vi "(Depricated) Nitrogen Feed Core.vi"() -> ()   [LabVIEW 2015]
doc: "Reads Storage Line State variable. Opens a single line."
panel:
  in  "error in (no error)":errorcluster
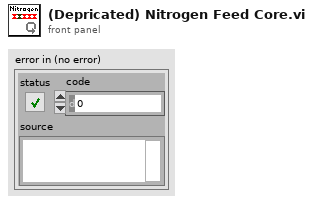
[diagram p1: front panel]
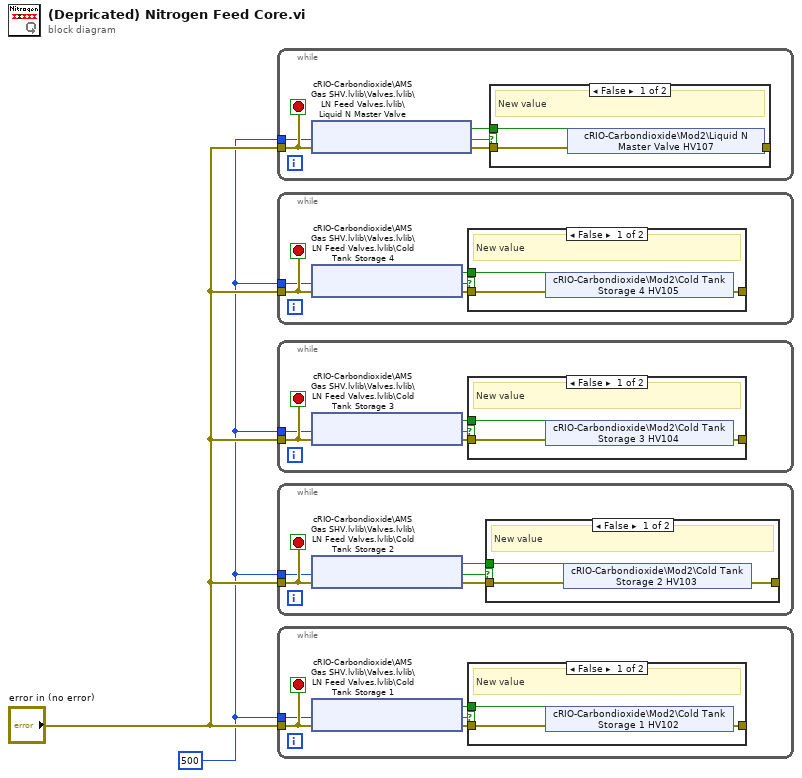
[diagram p0: block diagram]
diagram:
  w1 = 500 ("ms timeout (0)")
  n1 = while {
    tunnel: "error in (no error)" -> [w4]
    tunnel: w1 -> [w3]
    stop <- w4 stop-if-true
    n2 = shared-variable "cRIO-Carbondioxide\\AMS Gas SHV.lvlib\\Valves.lvlib\\LN Feed Valves.lvlib\\Liquid N Master Valve"(error in=w4, w3) -> (w5:bool, error out=w7:errorcluster, w6:bool)
    n3 = case shown="False" w6 {
      tunnel: w7 -> [w10 w11]
      tunnel: w5 -> [w9 _]
      tunnel: [w8 w11] -> _
      frame False {
        # "New value"
        n4 = shared-variable "cRIO-Carbondioxide\\Mod2\\Liquid N Master Valve HV107"(w9, error in=w10) -> (error out=w8:errorcluster)
      }
      frame True {
        # "Doing nothing"
        # "Timeout"
      }
    }
  }
  n5 = while {
    tunnel: "error in (no error)" -> [w13]
    tunnel: w1 -> [w12]
    stop <- w13 stop-if-true
    n6 = shared-variable "cRIO-Carbondioxide\\AMS Gas SHV.lvlib\\Valves.lvlib\\LN Feed Valves.lvlib\\Cold Tank Storage 4"(error in=w13, w12) -> (w14:bool, error out=w16:errorcluster, w15:bool)
    n7 = case shown="False" w15 {
      tunnel: w16 -> [w19 w20]
      tunnel: w14 -> [w18 _]
      tunnel: [w17 w20] -> _
      frame False {
        # "New value"
        n8 = shared-variable "cRIO-Carbondioxide\\Mod2\\Cold Tank Storage 4 HV105"(w18, error in=w19) -> (error out=w17:errorcluster)
      }
      frame True {
        # "Doing nothing"
        # "Timeout"
      }
    }
  }
  n9 = while {
    tunnel: "error in (no error)" -> [w22]
    tunnel: w1 -> [w21]
    stop <- w22 stop-if-true
    n10 = shared-variable "cRIO-Carbondioxide\\AMS Gas SHV.lvlib\\Valves.lvlib\\LN Feed Valves.lvlib\\Cold Tank Storage 3"(error in=w22, w21) -> (w23:bool, error out=w25:errorcluster, w24:bool)
    n11 = case shown="False" w24 {
      tunnel: w25 -> [w28 w29]
      tunnel: w23 -> [w27 _]
      tunnel: [w26 w29] -> _
      frame False {
        # "New value"
        n12 = shared-variable "cRIO-Carbondioxide\\Mod2\\Cold Tank Storage 3 HV104"(w27, error in=w28) -> (error out=w26:errorcluster)
      }
      frame True {
        # "Doing nothing"
        # "Timeout"
      }
    }
  }
  n13 = while {
    tunnel: "error in (no error)" -> [w31]
    tunnel: w1 -> [w30]
    stop <- w31 stop-if-true
    n14 = shared-variable "cRIO-Carbondioxide\\AMS Gas SHV.lvlib\\Valves.lvlib\\LN Feed Valves.lvlib\\Cold Tank Storage 2"(error in=w31, w30) -> (w32:bool, error out=w34:errorcluster, w33:bool)
    n15 = case shown="False" w33 {
      tunnel: w34 -> [w37 w38]
      tunnel: w32 -> [w36 _]
      tunnel: [w35 w38] -> _
      frame False {
        # "New value"
        n16 = shared-variable "cRIO-Carbondioxide\\Mod2\\Cold Tank Storage 2 HV103"(w36, error in=w37) -> (error out=w35:errorcluster)
      }
      frame True {
        # "Doing nothing"
        # "Timeout"
      }
    }
  }
  n17 = while {
    tunnel: "error in (no error)" -> [w40]
    tunnel: w1 -> [w39]
    stop <- w40 stop-if-true
    n18 = shared-variable "cRIO-Carbondioxide\\AMS Gas SHV.lvlib\\Valves.lvlib\\LN Feed Valves.lvlib\\Cold Tank Storage 1"(error in=w40, w39) -> (w41:bool, error out=w43:errorcluster, w42:bool)
    n19 = case shown="False" w42 {
      tunnel: w43 -> [w46 w47]
      tunnel: w41 -> [w45 _]
      tunnel: [w44 w47] -> _
      frame False {
        # "New value"
        n20 = shared-variable "cRIO-Carbondioxide\\Mod2\\Cold Tank Storage 1 HV102"(w45, error in=w46) -> (error out=w44:errorcluster)
      }
      frame True {
        # "Doing nothing"
        # "Timeout"
      }
    }
  }
